vi "1. Development Environment.vi"() -> ()   [LabVIEW 2014]
uses:
  ModuleA class/ModuleA.lvclass
  <vilib>/JKI/JKI SMO/SMO/Typedefs/SMOState --Enum.ctl
  <vilib>/JKI/JKI SMO/SMO/SMO.lvclass
panel:
  out "error out":errorcluster
  in  "error in (no error)":errorcluster
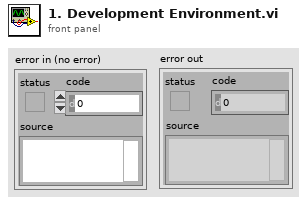
[diagram p1: front panel]
types:
  T1 = typedef "SMO.lvclass/Public Events.ctl" = cluster{"Error":refnum<user-event>, "State":refnum<user-event>, "Reserve State":refnum<user-event>}
  T2 = typedef "SMO.lvclass/SMOState --Enum.ctl" = enum16{"unknown", "Created", "Started", "Stopped"}
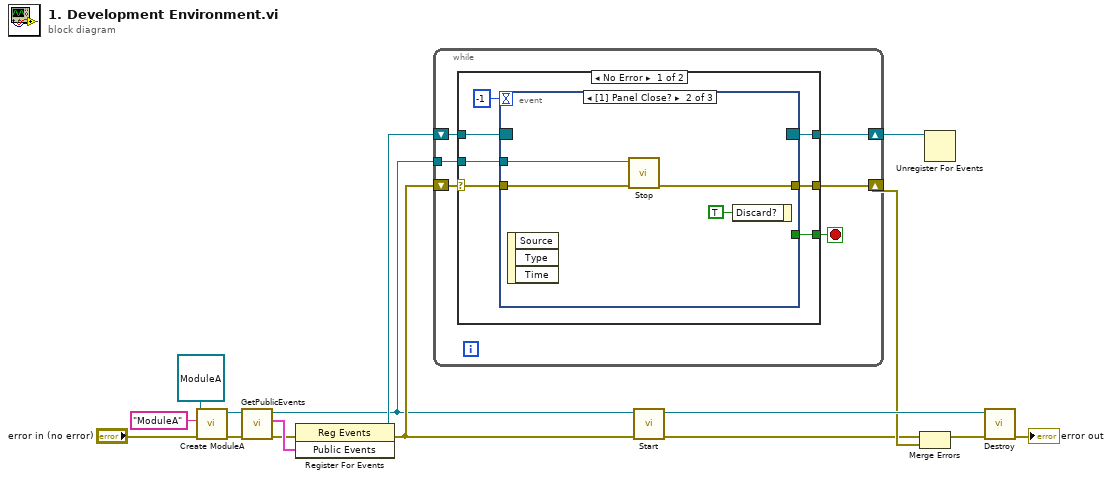
[diagram p0: block diagram]
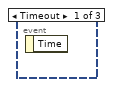
[diagram p2: hidden frame]
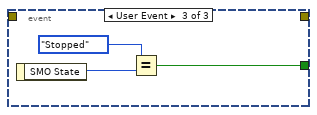
[diagram p3: hidden frame]
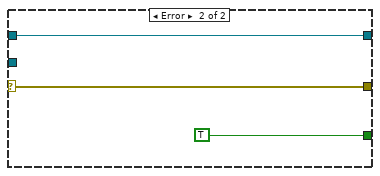
[diagram p4: hidden frame]
diagram:
  n1 = call "Create ModuleA.vi"("error in (no error)"="error in (no error)", "Subsystem Name (optional)"="ModuleA", "ModuleA in"=refnum<class "ModuleA.lvclass"> refnum ("ModuleA.lvclass")) -> ("error out"=w10:errorcluster, "ModuleA out"=w11:refnum<class "ModuleA.lvclass">)  [unwired: 6 in, 1 out]
  n2 = call <vilib>:"GetPublicEvents.vi"("error in (no error)"=w10, "SMO"=w11) -> ("error out"=w8:errorcluster, "Public Events"=w9:T1, "SMO out"=w1:refnum<class "ModuleA.lvclass">)  [unwired: 7 in]
  n3 = register-events(error in=w8, w9) -> (reference out=w7:refnum<event-registration>, error out=w6:errorcluster)  [unwired: 1 in]
  n4 = while {
    shift-right: [w21] -> w5
    shift-left: w7 -> [w22]
    shift-right: [w18] -> w4
    shift-left: w6 -> [w19]
    tunnel: w1 -> [w17]
    stop <- w20 stop-if-true
    n5 = case shown="No Error" w19 {
      selector: w19 -> [w24 w37]
      tunnel: w22 -> [w28 w39]
      tunnel: [w27 w39] -> w21
      tunnel: [w26 TRUE] -> w20
      tunnel: [w23 w37] -> w18
      tunnel: w17 -> [w25 _]
      frame No Error {
        n6 = event shown="[1] Panel Close?" {
          selector: w28 -> [_ _ _]
          dyn-events: [_ _ _] -> w27
          timeout: -1 -> [_ _ _]
          tunnel: [_ _ w34] -> w26
          tunnel: w25 -> [_ w33 _]
          tunnel: w24 -> [_ w32 _]
          tunnel: [_ w31 _] -> w23
          event Timeout {
            n7 = event-data() -> ()  [unwired: 1 in, 1 out]
          }
          event Panel Close? {
            n8 = event-data() -> ()  [unwired: 1 in, 3 out]
            n9 = call <vilib>:"Stop.vi"("error in (no error)"=w32, "SMO"=w33) -> ("error out"=w31:errorcluster)  [unwired: 8 in, 1 out]
            n10 = event-data("Discard?"=TRUE) -> ()  [unwired: 1 in, 1 out]
          }
          event User Event {
            n11 = event-data() -> ("SMO State"=w36:T2)  [unwired: 1 in]
            n12 = Equal?(x=SMOState_--Enum."Stopped", y=w36) -> (x = y?=w34:bool)
          }
        }
      }
      frame Error {
      }
    }
  }
  n13 = call <vilib>:"Start.vi"("error in (no error)"=w6, "SMO"=w1) -> ("error out"=w3:errorcluster, "SMO out"=w14:refnum<class "ModuleA.lvclass">)  [unwired: 8 in]
  n14 = Merge Errors(w3, w4) -> (w2:errorcluster)
  n15 = Unregister For Events(event registration refnum=w5) -> ()  [unwired: 1 in, 1 out]
  n16 = call <vilib>:"Destroy.vi"("error in (no error)"=w2, "SMO"=w14) -> ("error out"=→"error out":errorcluster)  [unwired: 9 in]
